vi "Initialize Resource Config-Ganging.vi"(8 "error in":errorcluster, 11 "Initialize Resource Config - Ganging":T1={"Master resource name "="", "Slave resource names"=[], "System configuration"=enum."Parallel", "Voltage/current level"=0.0, "Voltage/current level range"=0.0, "Limit symmetry"=enum."Symmetric", "Voltage/current limit range"=0.0, "Voltage/current limit low"=0.0, "Voltage/current limit high"=inf, "Output function"=1007, "Sense"=1009, "Transient response"=1038, "Voltage/current gain bandwith"=0.0, "Voltage/current compensation frequency"=0.0, "Voltage/current pole-zero ratio"=0.0, "DUT set-up time"=0.0} {"Transient response" items=["Slow"=1041, "Normal"=1038, "Fast"=1039, "Custom"=1042]; "Sense" items=["Local"=1008, "Remote"=1009]; "Output function" items=["DC Voltage"=1006, "DC Current"=1007, "Pulse Voltage"=1049, "Pulse Current"=1050]; "Voltage/current limit high" format="%#_6p"; "Voltage/current limit low" format="%#_6p"; "Voltage/current limit range" format="%#_6p"}) -> (0 "error out":errorcluster, 3 "Ganged Session Out":T2)   [LabVIEW 2021]
doc: "Initalize the source and load resource in ganging configuration."
uses:
  channel ganging/shared subVIs/ctl/NIDCPower_channel_ganging - ctl - ganged session.ctl
  channel ganging/shared subVIs/ctl/NIDCPower_channel_ganging - ctl - ganged config.ctl
  channel ganging/shared subVIs/ctl/NIDCPower_channel_ganging - ctl - channel mode.ctl
  controls/Initialize Resource Config-Ganging.ctl
  <instrlib>/niDCPower/nidcpower.llb/niDCPower Source Mode.ctl
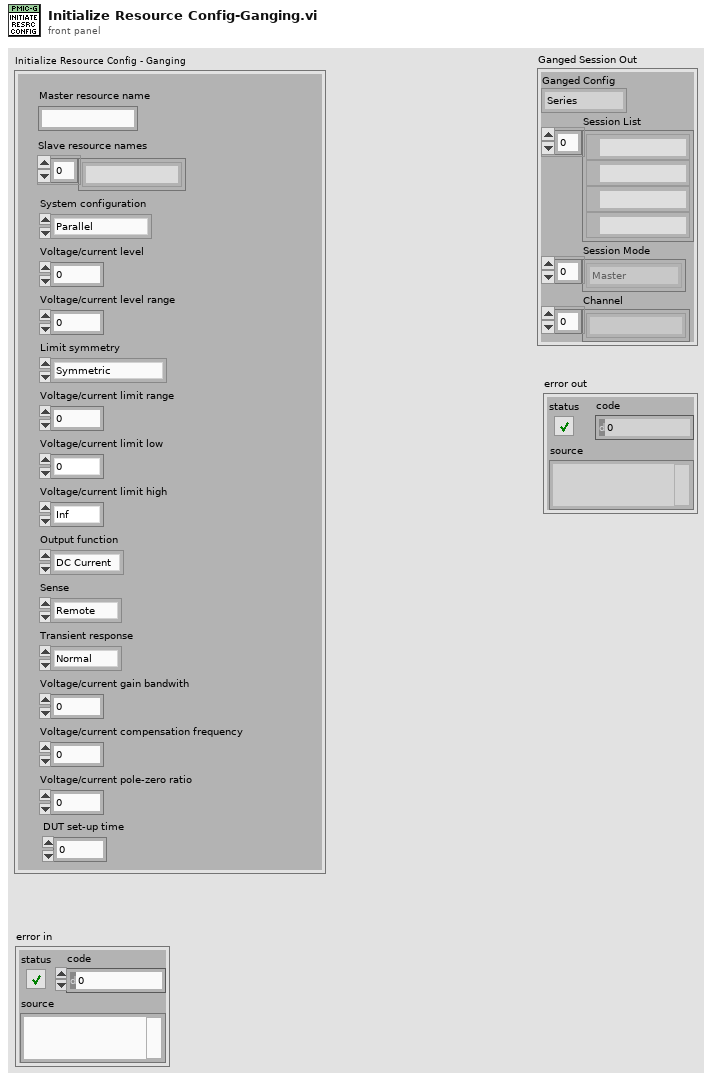
[diagram p1: front panel]
types:
  T1 = typedef "Initialize Resource Config-Ganging.ctl" = cluster{"Master resource name ":string, "Slave resource names":string[], "System configuration":enum32{"Series", "Parallel", "Manual"}, "Voltage/current level":dbl, "Voltage/current level range":dbl, "Limit symmetry":enum32{"Symmetric", "Asymmetric"}, "Voltage/current limit range":dbl, "Voltage/current limit low":dbl, "Voltage/current limit high":dbl, "Output function":i32, "Sense":i32, "Transient response":i32, "Voltage/current gain bandwith":dbl, "Voltage/current compensation frequency":dbl, "Voltage/current pole-zero ratio":dbl, "DUT set-up time":dbl}
  T2 = typedef "NIDCPower_channel_ganging - ctl - ganged session.ctl" = cluster{"Ganged Config":T3, "Session List":refnum<k15>[], "Session Mode":T4[], "Channel":string[]}
  T3 = typedef "NIDCPower_channel_ganging - ctl - ganged config.ctl" = enum32{"Series", "Parallel", "Manual"}
  T4 = typedef "NIDCPower_channel_ganging - ctl - channel mode.ctl" = enum32{"Master", "Slave", "Slave - Inverted"}
  T5 = typedef "niDCPower Source Mode.ctl" = i32
  T6 = typedef "NIDCPower_channel_ganging - ctl - channel def.ctl" = cluster{"resource name":refnum<k15>, "channels":string, "Channel Mode":T4}
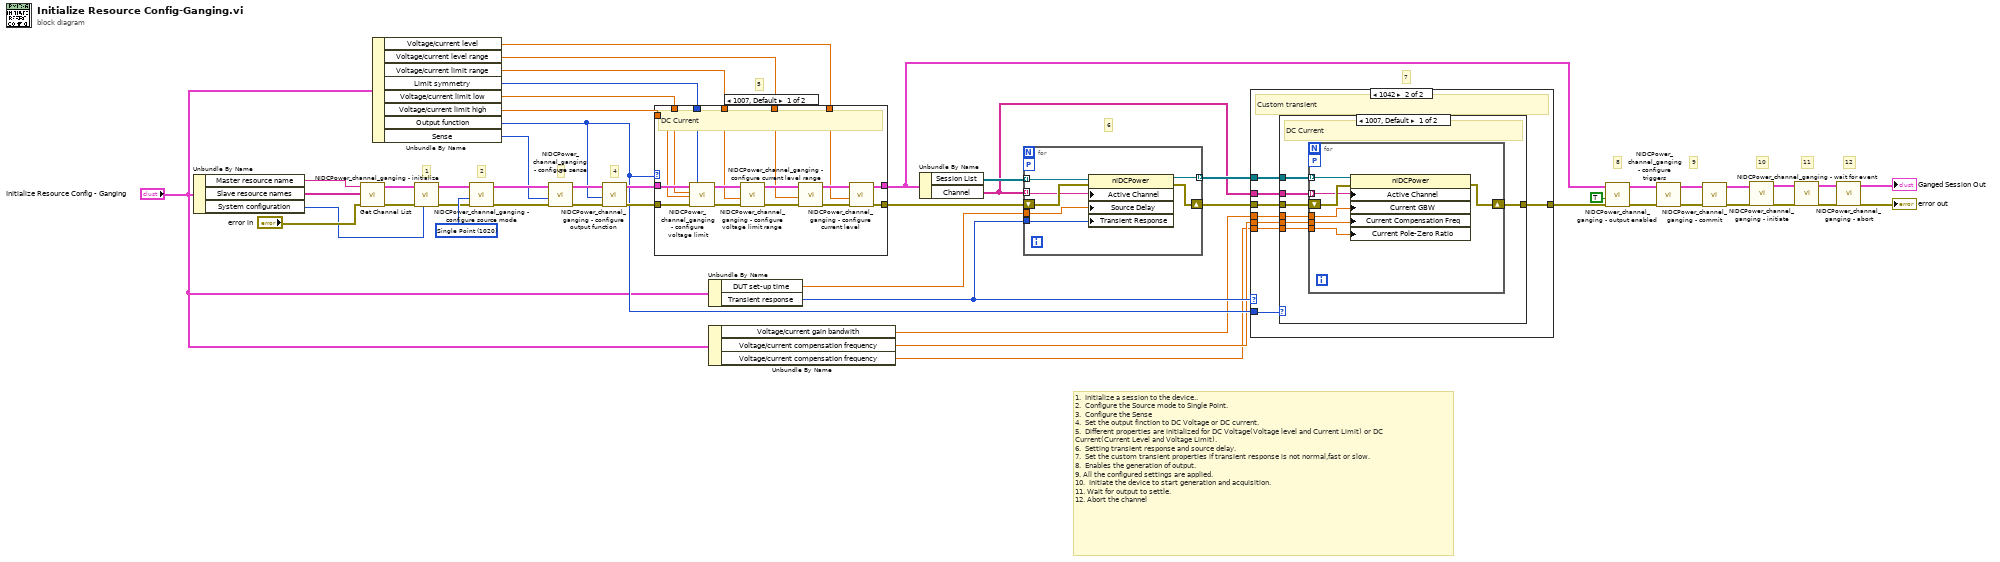
[diagram p0: block diagram]
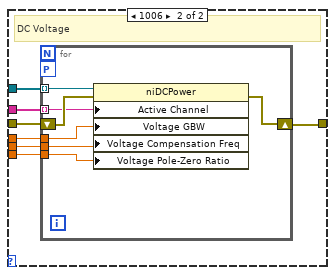
[diagram p3: hidden frame]
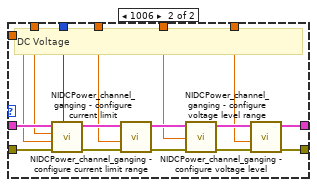
[diagram p4: hidden frame]
diagram:
  w43 = T5 1020 items=["Single Point"=1020, "Sequence"=1021] ("source mode")
  # "12"
  # "11"
  # "10"
  # "9"
  # "8"
  # "7"
  # "6"
  # "5"
  # "4"
  # "3"
  # "2"
  # "1"
  # "1.  Initialize a session to the device..\n2.  Configure the Source mode to Single Point.\n3.  Configure the Sense\n4.  Set the output finction to DC Voltage or DC current.\n5.  Different properties are initialized for DC Voltage(Voltage level and Current Limit) or DC Current(Current Level and Voltage Limit). \n6.  Setting transient response and source delay.\n7.  Set the custom transient properties if transient response is not normal,fast or slow.\n8.  Enables the generation of output.\n9. All the configured settings are applied.\n10.  Initiate the device to start generation and acquisition.\n11. Wait for output to settle.\n12. Abort the channel"
  n1 = Unbundle By Name("Initialize Resource Config - Ganging") -> ("Master resource name"=w49:string, "Slave resource names"=w48:string[], "System configuration"=w44:enum32{"Series", "Parallel", "Manual"})
  n2 = call "Get Channel List.vi"("error in (no error)"="error in", "Slave resource names"=w48, "Master resouce name"=w49) -> ("error out"=w45:errorcluster, "Channel List"=w46:T6[])  [unwired: 7 in]
  n3 = Unbundle By Name("Initialize Resource Config - Ganging") -> ("Voltage/current level"=w28:dbl, "Voltage/current level range"=w29:dbl, "Voltage/current limit range"=w30:dbl, "Limit symmetry"=w31:enum32{"Symmetric", "Asymmetric"}, "Voltage/current limit low"=w32:dbl, "Voltage/current limit high"=w33:dbl, "Output function"=w24:i32, "Sense"=w38:i32)
  n4 = call "NIDCPower_channel_ganging - initialize.vi"("Ganged Config"=w44, "error in (no error)"=w45, "Channel List"=w46) -> ("error out"=w42:errorcluster, "Ganged Session Out"=w41:T2)  [unwired: 7 in]
  n5 = call "NIDCPower_channel_ganging - configure source mode.vi"("error in (no error)"=w42, "source mode"=w43, "Ganged Session In"=w41) -> ("error out"=w39:errorcluster, "Ganged Session Out"=w40:T2)  [unwired: 7 in]
  n6 = call "NIDCPower_channel_ganging - configure sense.vi"("error in (no error)"=w39, "sense"=w38, "Ganged Session In"=w40) -> ("error out"=w37:errorcluster, "Ganged Session Out"=w36:T2)  [unwired: 7 in]
  n7 = call "NIDCPower_channel_ganging - configure output function.vi"("error in (no error)"=w37, "output function"=w24, "Ganged Session In"=w36) -> ("error out"=w34:errorcluster, "Ganged Session Out"=w35:T2)  [unwired: 7 in]
  n8 = case shown="1007, Default" w24 {
    tunnel: w35 -> [w59 w81]
    tunnel: w34 -> [w58 w77]
    tunnel: w33 -> [w57 w73]
    tunnel: w32 -> [w56 w72]
    tunnel: w31 -> [w55 w71]
    tunnel: w30 -> [w54 w70]
    tunnel: w29 -> [w53 w69]
    tunnel: w28 -> [w52 w68]
    tunnel: [w51 w67] -> w8
    tunnel: [w50 w66] -> w26
    frame 1007, Default {
      # "DC Current"
      n9 = call "NIDCPower_channel_ganging - configure voltage limit.vi"("Limit Symmetry"=w55, "error in (no error)"=w58, "voltage limit/hi"=w57, "voltage limit lo"=w56, "Ganged Session In"=w59) -> ("error out"=w65:errorcluster, "Ganged Session Out"=w64:T2)  [unwired: 5 in]
      n10 = call "NIDCPower_channel_ganging - configure voltage limit range.vi"("error in (no error)"=w65, "voltage level range"=w54, "Ganged Session In"=w64) -> ("error out"=w63:errorcluster, "Ganged Session Out"=w62:T2)  [unwired: 7 in]
      n11 = call "NIDCPower_channel_ganging - configure current level range.vi"("error in (no error)"=w63, "current level range"=w53, "Ganged Session In"=w62) -> ("error out"=w60:errorcluster, "Ganged Session Out"=w61:T2)  [unwired: 7 in]
      n12 = call "NIDCPower_channel_ganging - configure current level.vi"("error in (no error)"=w60, "current level"=w52, "Ganged Session In"=w61) -> ("error out"=w50:errorcluster, "Ganged Session Out"=w51:T2)  [unwired: 7 in]
    }
    frame 1006 {
      # "DC Voltage"
      n13 = call "NIDCPower_channel_ganging - configure current limit.vi"("Limit Symmetry"=w71, "error in (no error)"=w77, "Current limit/hi"=w73, "Current limit lo"=w72, "Ganged Session In"=w81) -> ("error out"=w76:errorcluster, "Ganged Session Out"=w80:T2)  [unwired: 5 in]
      n14 = call "NIDCPower_channel_ganging - configure current limit range.vi"("error in (no error)"=w76, "current limit range"=w70, "Ganged Session In"=w80) -> ("error out"=w75:errorcluster, "Ganged Session Out"=w79:T2)  [unwired: 7 in]
      n15 = call "NIDCPower_channel_ganging - configure voltage level range.vi"("error in (no error)"=w75, "voltage level range"=w69, "Ganged Session In"=w79) -> ("error out"=w74:errorcluster, "Ganged Session Out"=w78:T2)  [unwired: 7 in]
      n16 = call "NIDCPower_channel_ganging - configure voltage level.vi"("error in (no error)"=w74, "voltage level"=w68, "Ganged Session In"=w78) -> ("error out"=w66:errorcluster, "Ganged Session Out"=w67:T2)  [unwired: 7 in]
    }
  }
  n17 = Unbundle By Name("Initialize Resource Config - Ganging") -> ("DUT set-up time"=w6:dbl, "Transient response"=w25:i32)
  n18 = Unbundle By Name("Initialize Resource Config - Ganging") -> ("Voltage/current gain bandwith"=w4:dbl, "Voltage/current compensation frequency"=w3:dbl, "Voltage/current compensation frequency"=w2:dbl)
  n19 = Unbundle By Name(w8) -> ("Session List"=w27:refnum<k15>[], "Channel"=w21:string[])
  n20 = for {
    tunnel: w27 -> [w88] mode=indexing
    tunnel: w21 -> [w86] mode=indexing
    tunnel: w25 -> [w85]
    workers-P: _ -> [_]
    tunnel: [w84] -> w23 mode=indexing
    shift-right: [w83] -> w22
    shift-left: w26 -> [w87]
    tunnel: w6 -> [w82]
    n21 = property class="niDCPower"(reference=w88, error in=w87, "Active Channel"=w86, "Source Delay"=w82, "Transient Response"=w85) -> (reference out=w84:refnum<k15>, error out=w83:errorcluster)
  }
  n22 = case shown="1042" w25 {
    tunnel: w24 -> [_ w97]
    tunnel: w23 -> [_ w96]
    tunnel: w22 -> [w89 w95]
    tunnel: w21 -> [_ w94]
    tunnel: w4 -> [_ w93]
    tunnel: w3 -> [_ w92]
    tunnel: w2 -> [_ w91]
    tunnel: [w89 w90] -> w9
    frame Default {
    }
    frame 1042 {
      # "Custom transient"
      n23 = case shown="1007, Default" w97 {
        tunnel: w96 -> [w103 w118]
        tunnel: w95 -> [w104 w117]
        tunnel: w94 -> [w102 w116]
        tunnel: w93 -> [w101 w115]
        tunnel: w92 -> [w100 w114]
        tunnel: w91 -> [w99 w113]
        tunnel: [w98 w112] -> w90
        frame 1007, Default {
          # "DC Current"
          n24 = for {
            workers-P: _ -> [_]
            shift-right: [w109] -> w98
            shift-left: w104 -> [w110]
            tunnel: w103 -> [w111] mode=indexing
            tunnel: w102 -> [w108] mode=indexing
            tunnel: w101 -> [w107]
            tunnel: w100 -> [w106]
            tunnel: w99 -> [w105]
            n25 = property class="niDCPower"(reference=w111, error in=w110, "Active Channel"=w108, "Current GBW"=w107, "Current Compensation Freq"=w106, "Current Pole-Zero Ratio"=w105) -> (error out=w109:errorcluster)  [unwired: 1 out]
          }
        }
        frame 1006 {
          # "DC Voltage"
          n26 = for {
            workers-P: _ -> [_]
            tunnel: w118 -> [w125] mode=indexing
            shift-right: [w123] -> w112
            shift-left: w117 -> [w124]
            tunnel: w116 -> [w122] mode=indexing
            tunnel: w115 -> [w121]
            tunnel: w114 -> [w120]
            tunnel: w113 -> [w119]
            n27 = property class="niDCPower"(reference=w125, error in=w124, "Active Channel"=w122, "Voltage GBW"=w121, "Voltage Compensation Freq"=w120, "Voltage Pole-Zero Ratio"=w119) -> (error out=w123:errorcluster)  [unwired: 1 out]
          }
        }
      }
    }
  }
  n28 = call "NIDCPower_channel_ganging - output enabled.vi"("error in (no error)"=w9, "output enabled"=TRUE, "Ganged Session In"=w8) -> ("error out"=w20:errorcluster, "Ganged Session Out"=w19:T2)  [unwired: 7 in]
  n29 = call "NIDCPower_channel_ganging - configure triggers.vi"("error in (no error)"=w20, "Ganged Session In"=w19) -> ("error out"=w18:errorcluster, "Ganged Session Out"=w17:T2)  [unwired: 8 in]
  n30 = call "NIDCPower_channel_ganging - commit.vi"("error in (no error)"=w18, "Ganged Session In"=w17) -> ("error out"=w16:errorcluster, "Ganged Session Out"=w15:T2)  [unwired: 8 in]
  n31 = call "NIDCPower_channel_ganging - initiate.vi"("error in (no error)"=w16, "Ganged Session In"=w15) -> ("error out"=w14:errorcluster, "Ganged Session Out"=w13:T2)  [unwired: 8 in]
  n32 = call "NIDCPower_channel_ganging - wait for event.vi"("error in (no error)"=w14, "Ganged Session in"=w13) -> ("error out"=w12:errorcluster, "Ganged Session Out"=w11:T2)  [unwired: 8 in]
  n33 = call "NIDCPower_channel_ganging - abort.vi"("error in (no error)"=w12, "Ganged Session In"=w11) -> ("error out"=→"error out":errorcluster, "Ganged Session Out"=→"Ganged Session Out":T2)  [unwired: 8 in]
